vi "Sensor_Reads.vi"() -> ()   [LabVIEW 2018]
uses:
  Global_Variables/Drive_Globals.vi
  Global_Variables/Intake_Joint_Globals.vi
  Global_Variables/Elevator_Globals.vi
  Global_Variables/Climb_Globals.vi
  <vilib>/Rock Robotics/WPI/ThirdParty/Phoenix-LabVIEW/Pigeon IMU/CTRE_PigeonIMU_GetFusedHeading.vi
  Global_Variables/Sensor_Values.vi
  <vilib>/Rock Robotics/WPI/ThirdParty/Phoenix-LabVIEW/Motor Controller/Get/CTRE_Phoenix_MotorController_GetSelectedSensorData.vi
panel:
  out "Velocity_Front_Lift":i32
  out "Wheel_Speeds":T1(graph)
  out "Climb_IR_Rear":dbl
  out "Climb_IR_Rear":bool
  out "BL":i32
  out "FL":i32
  out "BR":i32
  out "FR":i32
  out "Climb_IR":bool
  in  "Over_Edge":dbl=0.8
  in  "y":i32=1000
  out "Ball_In":bool
  in  "Ball_Dist":dbl=1.9
  out "Intake_IR":dbl
  out "Elevator_Position":i32
  out "Joint_Position":i32
  out "Back_Climb_Position":i32
  out "Yaw_2":dbl
  out "Climb_IR":dbl
  out "Top_Joint_Limit":bool
  out "Bottom_Joint_Limit":bool
  out "Bottom_Elevator_Limit":bool
  out "Top_Elevator_Limit":bool
  out "Top_Climb_Limit_Front":bool
  out "Bottom_Climb_Limit_Front":bool
  out "Bottom_Climb_Limit_Back":bool
  out "Top_Climb_Limit_Back":bool
  out "Yaw_1":dbl
  out "Front Right Wheel":dbl
  out "Back Right Wheel":dbl
  out "Back Left Wheel":dbl
  out "Front Left Wheel":dbl
  out "Wheel_Pos":T2(graph)
  out "Front Right Wheel Drive":dbl
  out "Back Right Wheel Drive":dbl
  out "Back Left Wheel Drive":dbl
  out "Front Left Wheel Drive":dbl
  out "Front_Left_Wheel":bool
  out "Front_Right_Wheel":bool
  out "Back_Left_Wheel":bool
  out "Back_Right_Wheel":bool
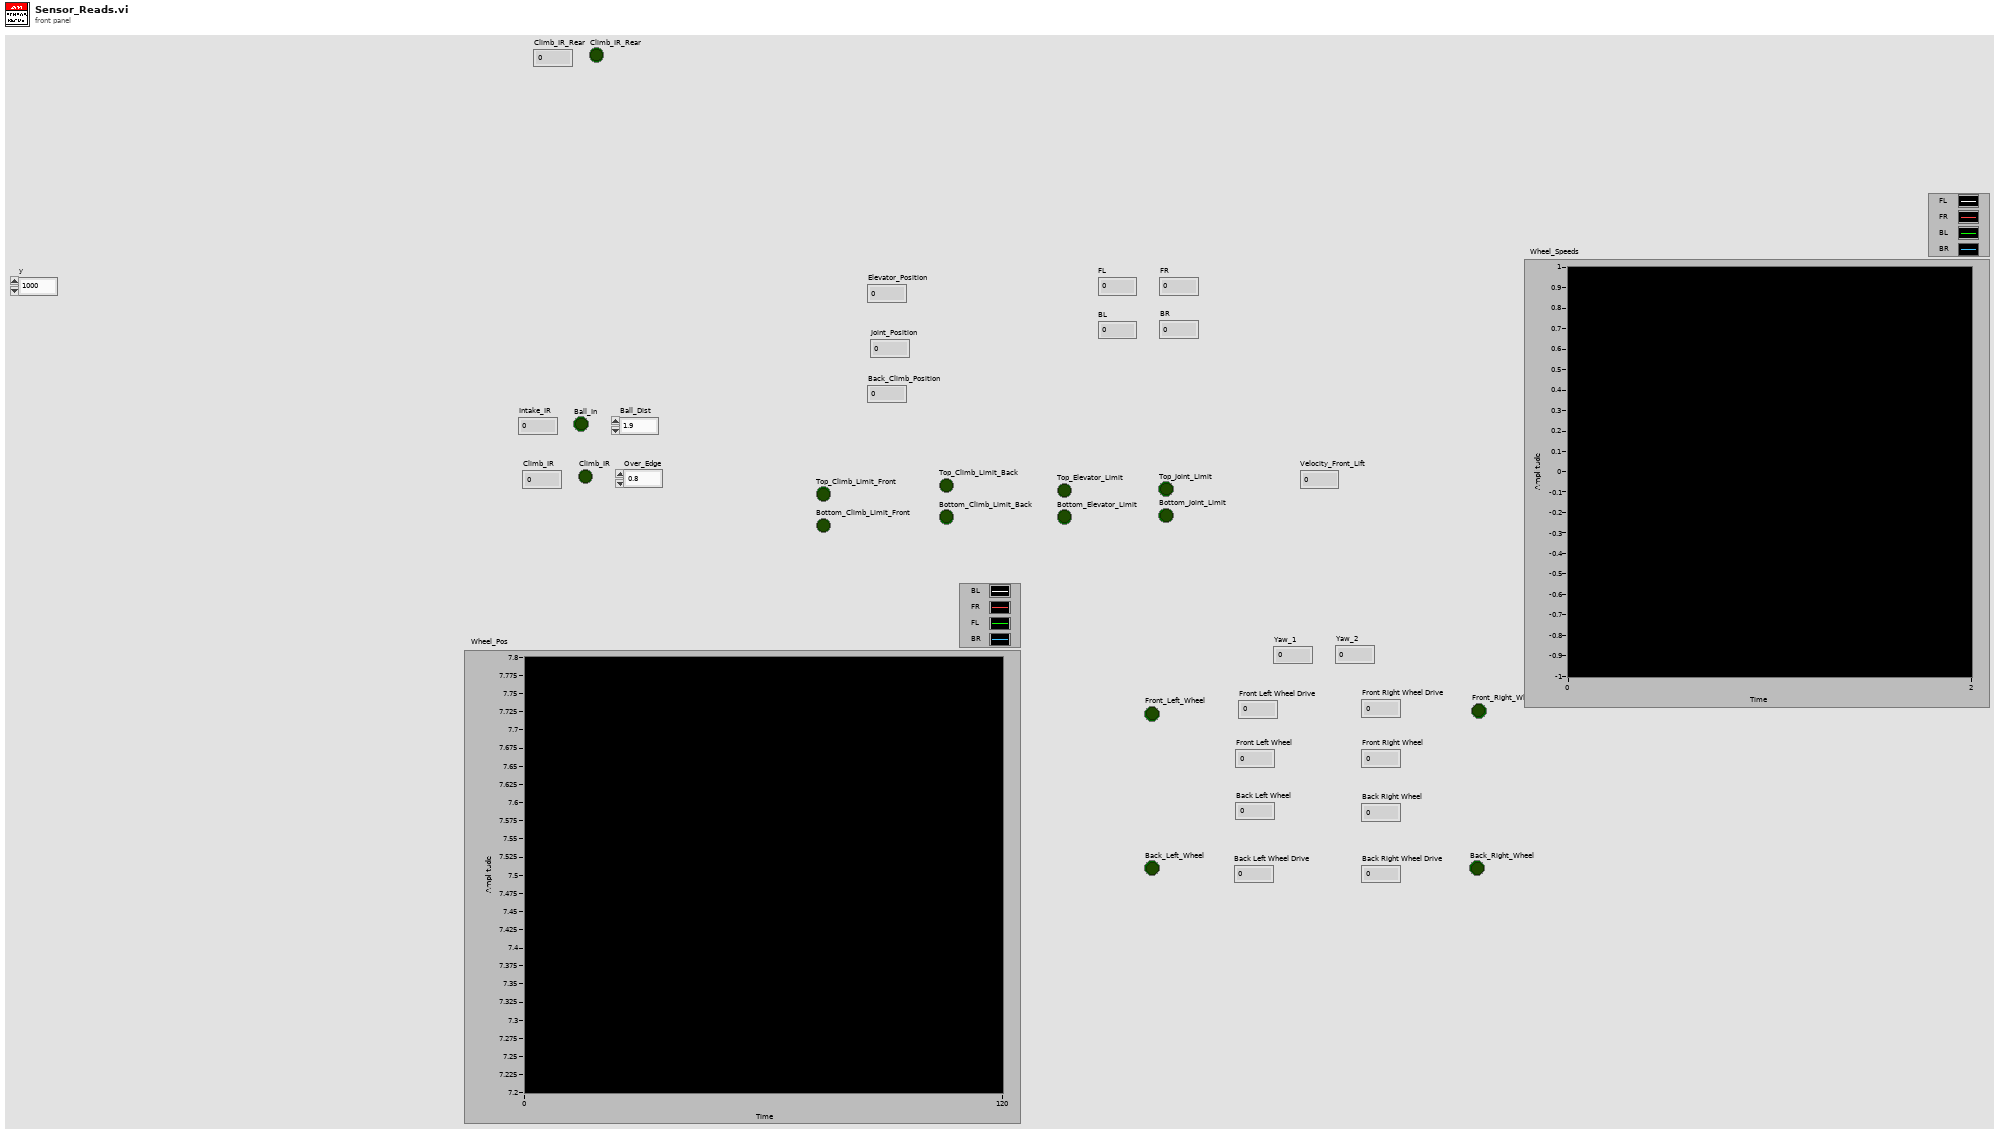
[diagram p1: front panel]
types:
  T1 = cluster{"Velocity (Raw Sensor Units per 100 ms)":i32, "Velocity (Raw Sensor Units per 100 ms)":i32, "Velocity (Raw Sensor Units per 100 ms)":i32, "Velocity (Raw Sensor Units per 100 ms)":i32}
  T2 = cluster{"Angle":dbl, "Angle":dbl, "Angle":dbl, "Angle":dbl}
  T3 = typedef "CTRE_PigeonIMU_DeviceRef.ctl" = cluster{"DeviceStatus":errorcluster, "Device Number":u8, "Type":T4, "Device ID":u32, "Handle":u64, "UsageFrame":u32, "Library Path":path}
  T4 = typedef "CTRE_PigeonIMU_ConnectionType.ctl" = u32
  T5 = typedef "WPI_MotorControlDeviceRef.ctl" = cluster{"DeviceStatus":errorcluster, "Type":T6, "PWM":cluster{"PWM Channel":T7, "DeadBand":T8}, "CAN":cluster{"Device Number":u8, "SetOutput VI Ref":variant, "GetOutput VI Ref":variant, "Enable VI Ref":variant, "Disable VI Ref":variant, "Data":variant}, "Invert":bool, "DIO PWM":cluster{"PWM \"Enable\" Channel":T7, "DIOChannel":T9, "PWM Rate":dbl}}
  T6 = typedef "WPI_MotorControlType.ctl" = enum16{"PWM", "CAN", "DIO PWM"}
  T7 = typedef "FPGA_DIOPWMChannel.ctl" = enum8{"PWM 0", "PWM 1", "PWM 2", "PWM 3", "PWM 4", "PWM 5", "PWM 6", "PWM 7", "PWM 8", "PWM 9", "PWM MXP 0", "PWM MXP 1", "PWM MXP 2", "PWM MXP 3", "PWM MXP 4", "PWM MXP 5", "PWM MXP 6", "PWM MXP 7", "PWM MXP 8", "PWM MXP 9", "Invalid"}
  T8 = typedef "WPI_PWMDeadband.ctl" = cluster{"Name":string, "maxPositivePwm":i32, "minPositivePwm":i32, "centerPwm":i32, "maxNegativePwm":i32, "minNegativePwm":i32, "angularRange":u16}
  T9 = typedef "FPGA_DIOChannel.ctl" = enum8{"DIO 0", "DIO 1", "DIO 2", "DIO 3", "DIO 4", "DIO 5", "DIO 6", "DIO 7", "DIO 8", "DIO 9", "DIO MXP 0", "DIO MXP 1", "DIO MXP 2", "DIO MXP 3", "DIO MXP 4", "DIO MXP 5", "DIO MXP 6", "DIO MXP 7", "DIO MXP 8", "DIO MXP 9", "DIO MXP 10", "DIO MXP 11", "DIO MXP 12", "DIO MXP 13", "DIO MXP 14", "DIO MXP 15", "SPI Port CS1", "SPI Port CS2", "SPI Port CS3", "SPI Port MISO", "SPI Port MOSI", "Invalid"}
  T10 = cluster{"Heading":dbl, "Valid?":bool, "Fusing?":bool}
  T11 = typedef "WPI_SwitchDevRef.ctl" = cluster{"DevStatus":errorcluster, "DIO Channel":T9, "CntIndex":T12, "Normally Closed":bool}
  T12 = typedef "FPGA_CounterCtrSystemIndex.ctl" = enum8{"Ctr 0", "Ctr 1", "Ctr 2", "Ctr 3", "Ctr 4", "Ctr 5", "Ctr 6", "Ctr 7", "Invalid"}
  T13 = typedef "WPI_AnalogChannelDevRef.ctl" = cluster{"DevStatus":errorcluster, "Analog Channel":T14}
  T14 = typedef "FPGA_AIChannel.ctl" = enum8{"AI 0", "AI 1", "AI 2", "AI 3", "AI MXP 0", "AI MXP 1", "AI MXP 2", "AI MXP 3", "Invalid"}
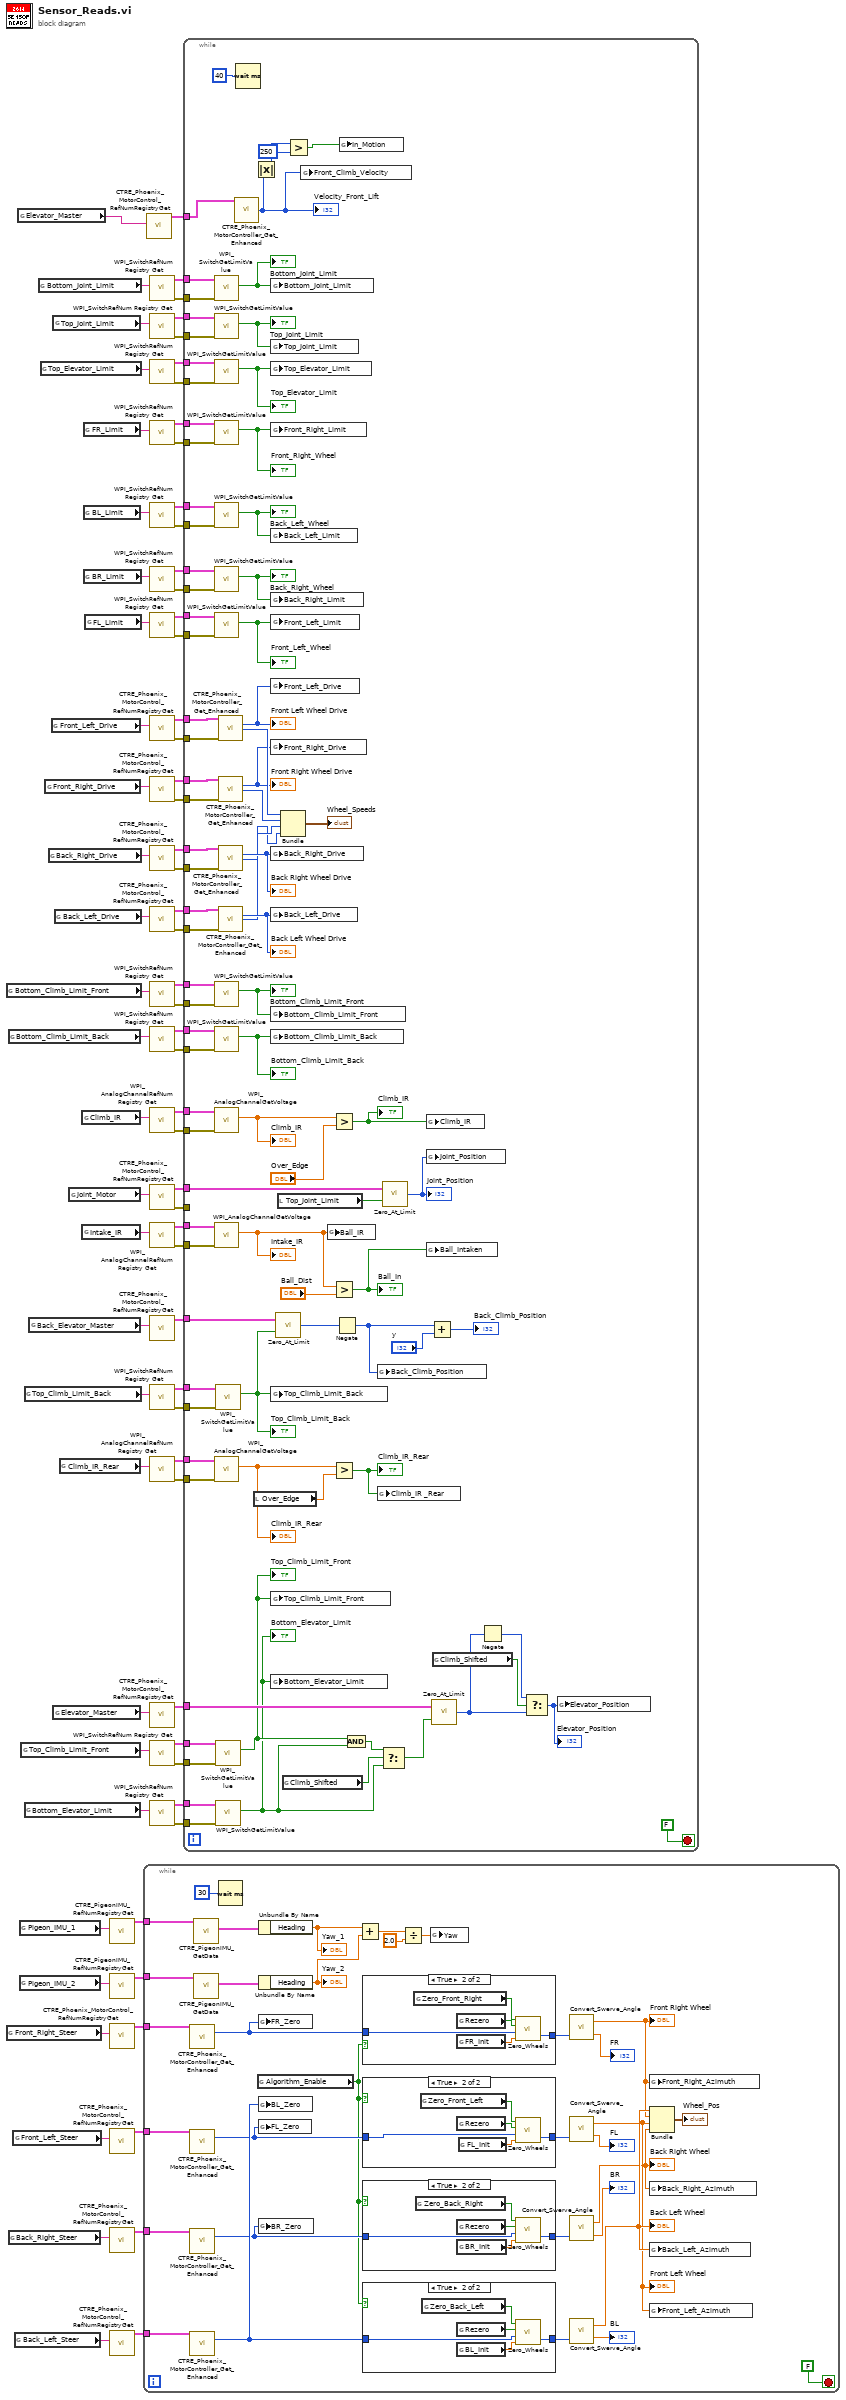
[diagram p0: block diagram]
diagram:
  n1 = global read "Elevator_Globals.vi" "Bottom_Climb_Limit_Front"() -> (w37:string)
  n2 = global read "Drive_Globals.vi" "Front_Right_Steer"() -> (w15:string)
  n3 = global read "Climb_Globals.vi" "Bottom_Climb_Limit_Back"() -> (w35:string)
  n4 = global read "Drive_Globals.vi" "Back_Right_Steer"() -> (w16:string)
  n5 = global read "Drive_Globals.vi" "Front_Left_Steer"() -> (w14:string)
  n6 = global read "Drive_Globals.vi" "Back_Left_Steer"() -> (w17:string)
  n7 = global read "Elevator_Globals.vi" "Elevator_Master"() -> (w2:string)
  n8 = global read "Drive_Globals.vi" "Pigeon_IMU_1"() -> (w8:string)
  n9 = global read "Drive_Globals.vi" "Pigeon_IMU_2"() -> (w9:string)
  n10 = global read "Elevator_Globals.vi" "Top_Climb_Limit_Front"() -> (w38:string)
  n11 = global read "Climb_Globals.vi" "Top_Climb_Limit_Back"() -> (w36:string)
  n12 = global read "Elevator_Globals.vi" "Bottom_Elevator_Limit"() -> (w39:string)
  n13 = global read "Climb_Globals.vi" "Back_Elevator_Master"() -> (w26:string)
  n14 = global read "Intake_Joint_Globals.vi" "Bottom_Joint_Limit"() -> (w41:string)
  n15 = global read "Elevator_Globals.vi" "Top_Elevator_Limit"() -> (w40:string)
  n16 = global read "Drive_Globals.vi" "Front_Right_Drive"() -> (w76:string)
  n17 = global read "Drive_Globals.vi" "Back_Right_Drive"() -> (w77:string)
  n18 = global read "Drive_Globals.vi" "Front_Left_Drive"() -> (w75:string)
  n19 = global read "Intake_Joint_Globals.vi" "Top_Joint_Limit"() -> (w42:string)
  n20 = global read "Elevator_Globals.vi" "Elevator_Master"() -> (w22:string)
  n21 = global read "Drive_Globals.vi" "Back_Left_Drive"() -> (w78:string)
  n22 = global read "Climb_Globals.vi" "Climb_IR_Rear"() -> (w5:string)
  n23 = global read "Intake_Joint_Globals.vi" "Joint_Motor"() -> (w23:string)
  n24 = global read "Climb_Globals.vi" "Climb_IR"() -> (w20:string)
  n25 = global read "Climb_Globals.vi" "Intake_IR"() -> (w28:string)
  n26 = global read "Drive_Globals.vi" "FR_Limit"() -> (w60:string)
  n27 = global read "Drive_Globals.vi" "BL_Limit"() -> (w61:string)
  n28 = global read "Drive_Globals.vi" "BR_Limit"() -> (w62:string)
  n29 = global read "Drive_Globals.vi" "FL_Limit"() -> (w59:string)
  n30 = call <vilib>:"CTRE_PigeonIMU_RefNumRegistryGet.vi"("refnum name"=w8) -> ("PigeonIMUDevRef"=w7:T3)  [unwired: 9 in, 1 out]
  n31 = call <vilib>:"CTRE_PigeonIMU_RefNumRegistryGet.vi"("refnum name"=w9) -> ("PigeonIMUDevRef"=w6:T3)  [unwired: 9 in, 1 out]
  n32 = call <vilib>:"CTRE_Phoenix_MotorControl_RefNumRegistryGet.vi"("refnum name"=w15) -> ("PhoenixMotorControlDevRef"=w12:T5)  [unwired: 9 in, 1 out]
  n33 = call <vilib>:"CTRE_Phoenix_MotorControl_RefNumRegistryGet.vi"("refnum name"=w14) -> ("PhoenixMotorControlDevRef"=w11:T5)  [unwired: 9 in, 1 out]
  n34 = call <vilib>:"CTRE_Phoenix_MotorControl_RefNumRegistryGet.vi"("refnum name"=w16) -> ("PhoenixMotorControlDevRef"=w10:T5)  [unwired: 9 in, 1 out]
  n35 = call <vilib>:"CTRE_Phoenix_MotorControl_RefNumRegistryGet.vi"("refnum name"=w17) -> ("PhoenixMotorControlDevRef"=w13:T5)  [unwired: 9 in, 1 out]
  n36 = while {
    tunnel: w13 -> [w94]
    tunnel: w12 -> [w95]
    tunnel: w11 -> [w109]
    tunnel: w10 -> [w108]
    tunnel: w7 -> [w101]
    tunnel: w6 -> [w100]
    stop <- FALSE stop-if-true
    n37 = call-poly <vilib>:"CTRE_Phoenix_MotorController_Get_Enhanced.vi"("PhoenixMotorControlDevRef"=w95) -> ("Position (Raw Sensor Units)"=w85:i32)  [unwired: 11 in, 3 out]
    n38 = call-poly <vilib>:"CTRE_Phoenix_MotorController_Get_Enhanced.vi"("PhoenixMotorControlDevRef"=w109) -> ("Position (Raw Sensor Units)"=w84:i32)  [unwired: 11 in, 3 out]
    n39 = call-poly <vilib>:"CTRE_Phoenix_MotorController_Get_Enhanced.vi"("PhoenixMotorControlDevRef"=w108) -> ("Position (Raw Sensor Units)"=w83:i32)  [unwired: 11 in, 3 out]
    n40 = call-poly <vilib>:"CTRE_Phoenix_MotorController_Get_Enhanced.vi"("PhoenixMotorControlDevRef"=w94) -> ("Position (Raw Sensor Units)"=w86:i32)  [unwired: 11 in, 3 out]
    n41 = call-poly <vilib>:"CTRE_PigeonIMU_GetData.vi"("PigeonIMUDevRef"=w101) -> ("Fused Heading"=w80:T10)  [unwired: 8 in, 2 out]
    n42 = call-poly <vilib>:"CTRE_PigeonIMU_GetData.vi"("PigeonIMUDevRef"=w100) -> ("Fused Heading"=w102:T10)  [unwired: 8 in, 2 out]
    n43 = Wait (ms)(milliseconds to wait=u32 30) -> ()  [unwired: 1 out]
    n44 = global read "Drive_Globals.vi" "Algorithm_Enable"() -> (w82:bool)
    n45 = Unbundle By Name(w80) -> ("Heading"=w96:dbl)
    "Yaw_1" <- w96
    n46 = Unbundle By Name(w102) -> ("Heading"=w81:dbl)
    "Yaw_2" <- w81
    n47 = global write "Drive_Globals.vi" "FR_Zero"(w85) -> ()
    n48 = global write "Drive_Globals.vi" "BL_Zero"(w86) -> ()
    n49 = global write "Drive_Globals.vi" "FL_Zero"(w84) -> ()
    n50 = global write "Drive_Globals.vi" "BR_Zero"(w83) -> ()
    n51 = Add(x=w96, y=w81) -> (x+y=w97:dbl)
    n52 = case shown="True" w82 {
      tunnel: [w124 w129] -> w90
      tunnel: w85 -> [w124 w128]
      frame False {
      }
      frame True {
        n53 = global read "Drive_Globals.vi" "Zero_Front_Right"() -> (w125:bool)
        n54 = global read "Sensor_Values.vi" "Rezero"() -> (w127:bool)
        n55 = global read "Drive_Globals.vi" "FR_Init"() -> (w126:dbl)
        n56 = call "Zero_Wheels.vi"("Init"=w126, "Encoder_In"=w128, "Re_Init"=w127, "Zero_Trigger"=w125) -> ("Encoder_Out"=w129:i32)  [unwired: 1 out]
      }
    }
    n57 = case shown="True" w82 {
      tunnel: [w118 w123] -> w93
      tunnel: w84 -> [w118 w122]
      frame False {
      }
      frame True {
        n58 = global read "Drive_Globals.vi" "Zero_Front_Left"() -> (w119:bool)
        n59 = global read "Sensor_Values.vi" "Rezero"() -> (w121:bool)
        n60 = global read "Drive_Globals.vi" "FL_Init"() -> (w120:dbl)
        n61 = call "Zero_Wheels.vi"("Init"=w120, "Encoder_In"=w122, "Re_Init"=w121, "Zero_Trigger"=w119) -> ("Encoder_Out"=w123:i32)  [unwired: 1 out]
      }
    }
    n62 = case shown="True" w82 {
      tunnel: w83 -> [w130 w135]
      tunnel: [w130 w134] -> w91
      frame False {
      }
      frame True {
        n63 = global read "Drive_Globals.vi" "Zero_Back_Right"() -> (w131:bool)
        n64 = global read "Sensor_Values.vi" "Rezero"() -> (w133:bool)
        n65 = global read "Drive_Globals.vi" "BR_Init"() -> (w132:dbl)
        n66 = call "Zero_Wheels.vi"("Init"=w132, "Encoder_In"=w135, "Re_Init"=w133, "Zero_Trigger"=w131) -> ("Encoder_Out"=w134:i32)  [unwired: 1 out]
      }
    }
    n67 = case shown="True" w82 {
      tunnel: w86 -> [w112 w117]
      tunnel: [w112 w116] -> w92
      frame False {
      }
      frame True {
        n68 = global read "Drive_Globals.vi" "Zero_Back_Left"() -> (w113:bool)
        n69 = global read "Sensor_Values.vi" "Rezero"() -> (w115:bool)
        n70 = global read "Drive_Globals.vi" "BL_Init"() -> (w114:dbl)
        n71 = call "Zero_Wheels.vi"("Init"=w114, "Encoder_In"=w117, "Re_Init"=w115, "Zero_Trigger"=w113) -> ("Encoder_Out"=w116:i32)  [unwired: 1 out]
      }
    }
    n72 = Divide(x=w97, y=2.0) -> (x/y=w99:dbl)
    n73 = global write "Sensor_Values.vi" "Yaw"(w99) -> ()
    n74 = call "Convert_Swerve_Angle.vi"("Current_Position (counts)"=w90) -> ("Unadjusted_Counts"=→"FR":dbl, "Angle"=w106:dbl)  [unwired: 2 in]
    "Front Right Wheel" <- w106
    n75 = call "Convert_Swerve_Angle.vi"("Current_Position (counts)"=w93) -> ("Unadjusted_Counts"=→"FL":dbl, "Angle"=w104:dbl)  [unwired: 2 in]
    "Front Left Wheel" <- w104
    n76 = call "Convert_Swerve_Angle.vi"("Current_Position (counts)"=w91) -> ("Unadjusted_Counts"=→"BR":dbl, "Angle"=w103:dbl)  [unwired: 2 in]
    "Back Right Wheel" <- w103
    n77 = call "Convert_Swerve_Angle.vi"("Current_Position (counts)"=w92) -> ("Unadjusted_Counts"=→"BL":dbl, "Angle"=w107:dbl)  [unwired: 2 in]
    "Back Left Wheel" <- w107
    n78 = global write "Sensor_Values.vi" "Front_Right_Azimuth"(w106) -> ()
    n79 = Bundle("Angle"=w107, "Angle"=w106, "Angle"=w104, "Angle"=w103) -> (→"Wheel_Pos":T2)  [unwired: 1 in]
    n80 = global write "Sensor_Values.vi" "Back_Right_Azimuth"(w103) -> ()
    n81 = global write "Sensor_Values.vi" "Back_Left_Azimuth"(w107) -> ()
    n82 = global write "Sensor_Values.vi" "Front_Left_Azimuth"(w104) -> ()
  }
  n83 = call <vilib>:"CTRE_Phoenix_MotorControl_RefNumRegistryGet.vi"("refnum name"=w2) -> ("PhoenixMotorControlDevRef"=w1:T5)  [unwired: 9 in, 1 out]
  n84 = call <vilib>:"WPI_SwitchRefNum Registry Get.vi"("refnum name"=w41) -> ("error out"=w43:errorcluster, "SwitchDevRef"=w44:T11)  [unwired: 9 in]
  n85 = call <vilib>:"WPI_SwitchRefNum Registry Get.vi"("refnum name"=w42) -> ("error out"=w45:errorcluster, "SwitchDevRef"=w46:T11)  [unwired: 9 in]
  n86 = call <vilib>:"WPI_SwitchRefNum Registry Get.vi"("refnum name"=w40) -> ("error out"=w47:errorcluster, "SwitchDevRef"=w48:T11)  [unwired: 9 in]
  n87 = call <vilib>:"WPI_SwitchRefNum Registry Get.vi"("refnum name"=w60) -> ("error out"=w64:errorcluster, "SwitchDevRef"=w63:T11)  [unwired: 9 in]
  n88 = call <vilib>:"WPI_SwitchRefNum Registry Get.vi"("refnum name"=w61) -> ("error out"=w66:errorcluster, "SwitchDevRef"=w65:T11)  [unwired: 9 in]
  n89 = call <vilib>:"WPI_SwitchRefNum Registry Get.vi"("refnum name"=w62) -> ("error out"=w67:errorcluster, "SwitchDevRef"=w68:T11)  [unwired: 9 in]
  n90 = call <vilib>:"WPI_SwitchRefNum Registry Get.vi"("refnum name"=w59) -> ("error out"=w69:errorcluster, "SwitchDevRef"=w70:T11)  [unwired: 9 in]
  n91 = call <vilib>:"CTRE_Phoenix_MotorControl_RefNumRegistryGet.vi"("refnum name"=w75) -> ("error out"=w32:errorcluster, "PhoenixMotorControlDevRef"=w72:T5)  [unwired: 9 in]
  n92 = call <vilib>:"CTRE_Phoenix_MotorControl_RefNumRegistryGet.vi"("refnum name"=w76) -> ("error out"=w33:errorcluster, "PhoenixMotorControlDevRef"=w73:T5)  [unwired: 9 in]
  n93 = call <vilib>:"CTRE_Phoenix_MotorControl_RefNumRegistryGet.vi"("refnum name"=w77) -> ("error out"=w31:errorcluster, "PhoenixMotorControlDevRef"=w71:T5)  [unwired: 9 in]
  n94 = call <vilib>:"CTRE_Phoenix_MotorControl_RefNumRegistryGet.vi"("refnum name"=w78) -> ("error out"=w34:errorcluster, "PhoenixMotorControlDevRef"=w74:T5)  [unwired: 9 in]
  n95 = call <vilib>:"WPI_SwitchRefNum Registry Get.vi"("refnum name"=w37) -> ("error out"=w51:errorcluster, "SwitchDevRef"=w52:T11)  [unwired: 9 in]
  n96 = call <vilib>:"WPI_SwitchRefNum Registry Get.vi"("refnum name"=w35) -> ("error out"=w57:errorcluster, "SwitchDevRef"=w56:T11)  [unwired: 9 in]
  n97 = call <vilib>:"WPI_AnalogChannelRefNum Registry Get.vi"("refnum name"=w20) -> ("error out"=w18:errorcluster, "AIDeviceRef"=w19:T13)  [unwired: 9 in]
  n98 = call <vilib>:"CTRE_Phoenix_MotorControl_RefNumRegistryGet.vi"("refnum name"=w23) -> ("error out"=w24:errorcluster, "PhoenixMotorControlDevRef"=w25:T5)  [unwired: 9 in]
  n99 = call <vilib>:"WPI_AnalogChannelRefNum Registry Get.vi"("refnum name"=w28) -> ("error out"=w29:errorcluster, "AIDeviceRef"=w30:T13)  [unwired: 9 in]
  n100 = call <vilib>:"CTRE_Phoenix_MotorControl_RefNumRegistryGet.vi"("refnum name"=w26) -> ("PhoenixMotorControlDevRef"=w27:T5)  [unwired: 9 in, 1 out]
  n101 = call <vilib>:"WPI_SwitchRefNum Registry Get.vi"("refnum name"=w36) -> ("error out"=w58:errorcluster, "SwitchDevRef"=w55:T11)  [unwired: 9 in]
  n102 = call <vilib>:"WPI_AnalogChannelRefNum Registry Get.vi"("refnum name"=w5) -> ("error out"=w3:errorcluster, "AIDeviceRef"=w4:T13)  [unwired: 9 in]
  n103 = call <vilib>:"CTRE_Phoenix_MotorControl_RefNumRegistryGet.vi"("refnum name"=w22) -> ("PhoenixMotorControlDevRef"=w21:T5)  [unwired: 9 in, 1 out]
  n104 = call <vilib>:"WPI_SwitchRefNum Registry Get.vi"("refnum name"=w38) -> ("error out"=w53:errorcluster, "SwitchDevRef"=w54:T11)  [unwired: 9 in]
  n105 = call <vilib>:"WPI_SwitchRefNum Registry Get.vi"("refnum name"=w39) -> ("error out"=w49:errorcluster, "SwitchDevRef"=w50:T11)  [unwired: 9 in]
  n106 = while {
    tunnel: w74 -> [w224]
    tunnel: w73 -> [w223]
    tunnel: w72 -> [w222]
    tunnel: w71 -> [w221]
    tunnel: w70 -> [w220]
    tunnel: w69 -> [w219]
    tunnel: w68 -> [w218]
    tunnel: w67 -> [w217]
    tunnel: w66 -> [w216]
    tunnel: w65 -> [w215]
    tunnel: w64 -> [w214]
    tunnel: w63 -> [w213]
    tunnel: w58 -> [w205]
    tunnel: w57 -> [w208]
    tunnel: w56 -> [w207]
    tunnel: w55 -> [w206]
    tunnel: w54 -> [w201]
    tunnel: w53 -> [w200]
    tunnel: w52 -> [w203]
    tunnel: w51 -> [w202]
    tunnel: w50 -> [w199]
    tunnel: w49 -> [w198]
    tunnel: w48 -> [w197]
    tunnel: w47 -> [w196]
    tunnel: w46 -> [w192]
    tunnel: w45 -> [w191]
    tunnel: w44 -> [w190]
    tunnel: w43 -> [w189]
    tunnel: w34 -> [w188]
    tunnel: w33 -> [w187]
    tunnel: w32 -> [w186]
    tunnel: w31 -> [w185]
    tunnel: w30 -> [w184]
    tunnel: w29 -> [w183]
    tunnel: w27 -> [w178]
    tunnel: w25 -> [w162]
    tunnel: w24 -> [_]
    tunnel: w21 -> [w179]
    tunnel: w19 -> [w181]
    tunnel: w18 -> [w180]
    tunnel: w4 -> [w158]
    tunnel: w3 -> [w157]
    tunnel: w1 -> [w145]
    stop <- FALSE stop-if-true
    n107 = call <vilib>:"WPI_SwitchGetLimitValue.vi"("error in (no error)"=w189, "SwitchDevRef"=w190) -> ("Switch Pressed"=w194:bool)  [unwired: 7 in, 2 out]
    "Bottom_Joint_Limit" <- w194
    n108 = call <vilib>:"WPI_SwitchGetLimitValue.vi"("error in (no error)"=w191, "SwitchDevRef"=w192) -> ("Switch Pressed"=w193:bool)  [unwired: 7 in, 2 out]
    "Top_Joint_Limit" <- w193
    n109 = call <vilib>:"WPI_SwitchGetLimitValue.vi"("error in (no error)"=w196, "SwitchDevRef"=w197) -> ("Switch Pressed"=w182:bool)  [unwired: 7 in, 2 out]
    "Top_Elevator_Limit" <- w182
    n110 = call <vilib>:"WPI_SwitchGetLimitValue.vi"("error in (no error)"=w214, "SwitchDevRef"=w213) -> ("Switch Pressed"=w211:bool)  [unwired: 7 in, 2 out]
    "Front_Right_Wheel" <- w211
    n111 = call <vilib>:"WPI_SwitchGetLimitValue.vi"("error in (no error)"=w216, "SwitchDevRef"=w215) -> ("Switch Pressed"=w210:bool)  [unwired: 7 in, 2 out]
    "Back_Left_Wheel" <- w210
    n112 = call <vilib>:"WPI_SwitchGetLimitValue.vi"("error in (no error)"=w217, "SwitchDevRef"=w218) -> ("Switch Pressed"=w209:bool)  [unwired: 7 in, 2 out]
    "Back_Right_Wheel" <- w209
    n113 = call <vilib>:"WPI_SwitchGetLimitValue.vi"("error in (no error)"=w219, "SwitchDevRef"=w220) -> ("Switch Pressed"=w212:bool)  [unwired: 7 in, 2 out]
    "Front_Left_Wheel" <- w212
    n114 = call <vilib>:"WPI_SwitchGetLimitValue.vi"("error in (no error)"=w202, "SwitchDevRef"=w203) -> ("Switch Pressed"=w195:bool)  [unwired: 7 in, 2 out]
    "Bottom_Climb_Limit_Front" <- w195
    n115 = call <vilib>:"WPI_SwitchGetLimitValue.vi"("error in (no error)"=w208, "SwitchDevRef"=w207) -> ("Switch Pressed"=w204:bool)  [unwired: 7 in, 2 out]
    "Bottom_Climb_Limit_Back" <- w204
    n116 = call <vilib>:"WPI_AnalogChannelGetVoltage.vi"("error in (no error)"=w180, "AIDeviceRef"=w181) -> ("Voltage"=w163:dbl)  [unwired: 7 in, 2 out]
    "Climb_IR" <- w163
    n117 = call <vilib>:"WPI_AnalogChannelGetVoltage.vi"("error in (no error)"=w183, "AIDeviceRef"=w184) -> ("Voltage"=w146:dbl)  [unwired: 7 in, 2 out]
    "Intake_IR" <- w146
    n118 = call <vilib>:"WPI_AnalogChannelGetVoltage.vi"("error in (no error)"=w157, "AIDeviceRef"=w158) -> ("Voltage"=w159:dbl)  [unwired: 7 in, 2 out]
    "Climb_IR_Rear" <- w159
    n119 = call <vilib>:"WPI_SwitchGetLimitValue.vi"("error in (no error)"=w205, "SwitchDevRef"=w206) -> ("Switch Pressed"=w177:bool)  [unwired: 7 in, 2 out]
    "Top_Climb_Limit_Back" <- w177
    n120 = call <vilib>:"WPI_SwitchGetLimitValue.vi"("error in (no error)"=w200, "SwitchDevRef"=w201) -> ("Switch Pressed"=w137:bool)  [unwired: 7 in, 2 out]
    "Top_Climb_Limit_Front" <- w137
    n121 = call <vilib>:"WPI_SwitchGetLimitValue.vi"("error in (no error)"=w198, "SwitchDevRef"=w199) -> ("Switch Pressed"=w136:bool)  [unwired: 7 in, 2 out]
    "Bottom_Elevator_Limit" <- w136
    n122 = call-poly <vilib>:"CTRE_Phoenix_MotorController_Get_Enhanced.vi"("PhoenixMotorControlDevRef"=w222, "error in"=w186) -> ("Position (Raw Sensor Units)"=w154:i32, "Velocity (Raw Sensor Units per 100 ms)"=w153:i32)  [unwired: 10 in, 2 out]
    "Front Left Wheel Drive" <- w154
    n123 = call-poly <vilib>:"CTRE_Phoenix_MotorController_Get_Enhanced.vi"("PhoenixMotorControlDevRef"=w223, "error in"=w187) -> ("Position (Raw Sensor Units)"=w150:i32, "Velocity (Raw Sensor Units per 100 ms)"=w152:i32)  [unwired: 10 in, 2 out]
    "Front Right Wheel Drive" <- w150
    n124 = call-poly <vilib>:"CTRE_Phoenix_MotorController_Get_Enhanced.vi"("PhoenixMotorControlDevRef"=w221, "error in"=w185) -> ("Position (Raw Sensor Units)"=w149:i32, "Velocity (Raw Sensor Units per 100 ms)"=w139:i32)  [unwired: 10 in, 2 out]
    "Back Right Wheel Drive" <- w149
    n125 = call-poly <vilib>:"CTRE_Phoenix_MotorController_Get_Enhanced.vi"("PhoenixMotorControlDevRef"=w224, "error in"=w188) -> ("Position (Raw Sensor Units)"=w148:i32, "Velocity (Raw Sensor Units per 100 ms)"=w140:i32)  [unwired: 10 in, 2 out]
    "Back Left Wheel Drive" <- w148
    n126 = call-poly <vilib>:"CTRE_Phoenix_MotorController_Get_Enhanced.vi"("PhoenixMotorControlDevRef"=w145) -> ("Velocity (Raw Sensor Units per 100 ms)"=w144:i32)  [unwired: 11 in, 3 out]
    "Velocity_Front_Lift" <- w144
    n127 = Wait (ms)(milliseconds to wait=u32 40) -> ()  [unwired: 1 out]
    n128 = local read "Over_Edge"() -> (w156:dbl)
    n129 = Absolute Value(x=w144) -> (abs(x)=w141:i32)
    n130 = global write "Sensor_Values.vi" "Bottom_Joint_Limit"(w194) -> ()
    n131 = global write "Sensor_Values.vi" "Top_Joint_Limit"(w193) -> ()
    n132 = global write "Sensor_Values.vi" "Top_Elevator_Limit"(w182) -> ()
    n133 = global write "Sensor_Values.vi" "Front_Right_Limit"(w211) -> ()
    n134 = global write "Sensor_Values.vi" "Back_Left_Limit"(w210) -> ()
    n135 = global write "Sensor_Values.vi" "Back_Right_Limit"(w209) -> ()
    n136 = global write "Sensor_Values.vi" "Front_Left_Limit"(w212) -> ()
    n137 = global write "Sensor_Values.vi" "Front_Left_Drive"(w154) -> ()
    n138 = global write "Sensor_Values.vi" "Front_Right_Drive"(w150) -> ()
    n139 = global write "Sensor_Values.vi" "Back_Right_Drive"(w149) -> ()
    n140 = global write "Sensor_Values.vi" "Back_Left_Drive"(w148) -> ()
    n141 = global write "Sensor_Values.vi" "Bottom_Climb_Limit_Front"(w195) -> ()
    n142 = global write "Sensor_Values.vi" "Bottom_Climb_Limit_Back"(w204) -> ()
    n143 = global write "Sensor_Values.vi" "Top_Climb_Limit_Back"(w177) -> ()
    n144 = global write "Sensor_Values.vi" "Top_Climb_Limit_Front"(w137) -> ()
    n145 = global write "Sensor_Values.vi" "Bottom_Elevator_Limit"(w136) -> ()
    n146 = call "Zero_At_Limit.vi"("Limit_Hit"=w177, "Talon_Ref_In"=w178) -> ("Sensor_Out"=w175:i32)
    n147 = local read "Top_Joint_Limit"() -> (w160:bool)
    n148 = Bundle("Velocity (Raw Sensor Units per 100 ms)"=w153, "Velocity (Raw Sensor Units per 100 ms)"=w152, "Velocity (Raw Sensor Units per 100 ms)"=w140, "Velocity (Raw Sensor Units per 100 ms)"=w139) -> (→"Wheel_Speeds":T1)  [unwired: 1 in]
    n149 = global read "Elevator_Globals.vi" "Climb_Shifted"() -> (w173:bool)
    n150 = Greater?(x=w141, y=250) -> (0:w142:bool)
    n151 = global write "Sensor_Values.vi" "Front_Climb_Velocity"(w144) -> ()
    n152 = global write "Sensor_Values.vi" "Ball_IR"(w146) -> ()
    n153 = Greater?(x=w163, y="Over_Edge") -> (0:w165:bool)
    "Climb_IR" <- w165
    n154 = Greater?(x=w146, y="Ball_Dist") -> (0:w147:bool)
    "Ball_In" <- w147
    n155 = Greater?(x=w159, y=w156) -> (0:w155:bool)
    "Climb_IR_Rear" <- w155
    n156 = Negate(x=w175) -> (-x=w172:i32)
    n157 = global write "Sensor_Values.vi" "In_Motion"(w142) -> ()
    n158 = And(x=w137, y=w136) -> (x .and. y?=w138:bool)
    n159 = global write "Sensor_Values.vi" "Back_Climb_Position"(w172) -> ()
    n160 = global write "Sensor_Values.vi" "Climb_IR _Rear"(w155) -> ()
    n161 = Select(t=w138, s=w173, f=w136) -> (s? t:f=w174:bool)
    n162 = call "Zero_At_Limit.vi"("Limit_Hit"=w160, "Talon_Ref_In"=w162) -> ("Sensor_Out"=w161:i32)
    "Joint_Position" <- w161
    n163 = global write "Sensor_Values.vi" "Climb_IR"(w165) -> ()
    n164 = global write "Sensor_Values.vi" "Joint_Position"(w161) -> ()
    n165 = global write "Sensor_Values.vi" "Ball_Intaken"(w147) -> ()
    n166 = Add(x=w172, y="y") -> (x+y=→"Back_Climb_Position":i32)
    n167 = call "Zero_At_Limit.vi"("Limit_Hit"=w174, "Talon_Ref_In"=w179) -> ("Sensor_Out"=w166:i32)
    n168 = global read "Elevator_Globals.vi" "Climb_Shifted"() -> (w167:bool)
    n169 = Negate(x=w166) -> (-x=w169:i32)
    n170 = Select(t=w169, s=w167, f=w166) -> (s? t:f=w168:i32)
    "Elevator_Position" <- w168
    n171 = global write "Sensor_Values.vi" "Elevator_Position"(w168) -> ()
  }
